vi "Read Attribute (U32).vi"(8 "error in":errorcluster, 9 "default":u32, 10 "Attribute Name":string, 11 "node in":refnum<k20>) -> (0 "error out":errorcluster, 1 "value":u32, 3 "node out":refnum<k20>)   [LabVIEW 2020, in "AIM ARINC 664 Import.lvlib"]
uses:
  AIM ARINC 664 Import.lvlib
  <resource>/objmgr/DOMUserDefRef.rc
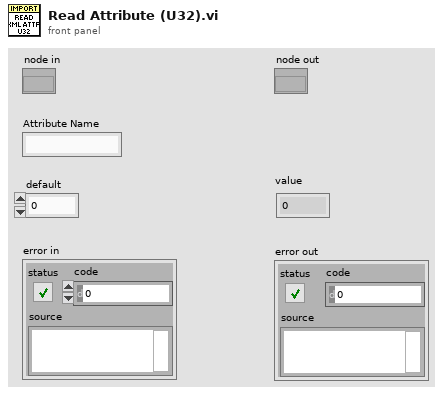
[diagram p1: front panel]
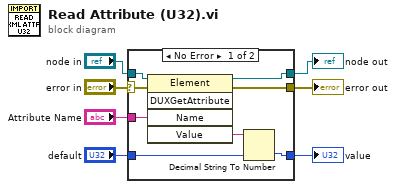
[diagram p0: block diagram]
diagram:
  n1 = case shown="No Error" "error in" {
    selector: "error in" -> [w8 w18]
    tunnel: [w9 w18] -> w7
    tunnel: "node in" -> [w14 w17]
    tunnel: "Attribute Name" -> [w15 _]
    tunnel: [w10 w16] -> w4
    tunnel: [w13 w17] -> w3
    tunnel: "default" -> [w11 w16]
    frame No Error {
      n2 = invoke class="Element" method="DUXGetAttribute"(reference=w14, error in=w8, "Name"=w15) -> (reference out=w13:refnum<k20>, error out=w9:errorcluster, "Value"=w12:string)  [unwired: 2 in, 2 out]
      n3 = Decimal String To Number(string=w12, default (0L)=w11) -> (number=w10:u32)  [unwired: 1 in, 1 out]
    }
    frame Error {
    }
  }
  "error out" <- w7
  "node out" <- w3
  "value" <- w4
